vi "Create point.vi"(2 "Colour":T1={"Red"=1.0, "Green"=1.0, "Blue"=1.0, "Alpha"=1.0}, 3 "Point size":dbl=3.0, 4 "Point":sgl[](array[numeric])=[0.0, 0.0, 0.0]) -> (0 "Error out":errorcluster, 1 "Point out":refnum<vi>)   [LabVIEW 2017]
uses:
  <vilib>/Utility/miscctls.llb/LVRGBAColorTypeDef.ctl
  <vilib>/Utility/miscctls.llb/LV3DPointTypeDef.ctl
  <vilib>/picture/3D Picture Control/Object/Create Object (drawable).vi
  <vilib>/picture/3D Picture Control/NI_3D Picture Control.lvlib
panel:
  # "PN 23/10/17"
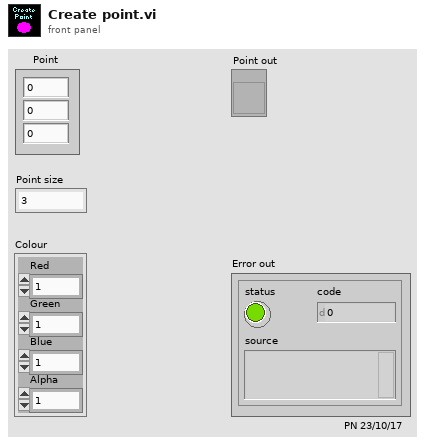
[diagram p1: front panel]
types:
  T1 = typedef "LVRGBAColorTypeDef.ctl" = cluster{"Red":sgl, "Green":sgl, "Blue":sgl, "Alpha":sgl}
  T2 = enum16{"Inherit Value", "Points", "Wireframe", "Polygons"}
  T3 = typedef "LV3DPointTypeDef.ctl" = cluster{"X":sgl, "Y":sgl, "Z":sgl}
  T4 = enum16{"Inherit Material", "Use entire Material", "Ignore Ambient", "Ignore Diffuse", "Ignore Specular", "Ignore Emission", "Ignore Ambient and Diffuse"}
  T5 = enum16{"Overall", "Per Primitive", "Per Vertex", "Binding Off"}
  T6 = enum16{"Points", "Lines", "Line Strip", "Line Loop", "Triangles", "Triangle Strip", "Triangle Fan", "Quads", "Quad Strip", "Polygon"}
  T7 = enum16{"Inherit Value", "No Culling", "Cull Back Face", "Cull Front Face", "Cull Both Faces"}
  T8 = enum16{"Inherit Value", "Counterclockwise", "Clockwise"}
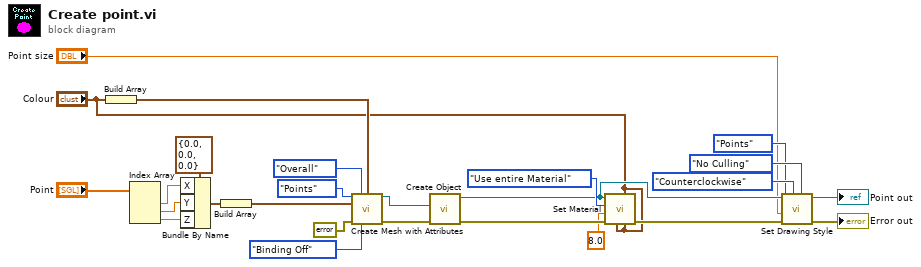
[diagram p0: block diagram]
diagram:
  n1 = Build Array("Colour") -> (w9:T1[])
  n2 = Index Array(array="Point") -> (element #1=w6:sgl, element #2=w5:sgl, element #3=w4:sgl)  [unwired: 3 in]
  n3 = Bundle By Name(cluster=T3 {"X"=0.0, "Y"=0.0, "Z"=0.0} ("3D Point"), "X"=w6, "Y"=w5, "Z"=w4) -> (w19:T3)
  n4 = Build Array(w19) -> (w2:T3[])
  n5 = call <vilib>:"Create Mesh with Attributes.vi"("Draw Mode"=T6."Points", "Color Binding Mode"=T5."Overall", "Color Array"=w9, "Vertex Array"=w2, "error in (no error)"=errorcluster {"status"=FALSE, "code"=0, "source"=""}, "Normal Binding Mode"=T5."Binding Off") -> ("New Mesh Refnum"=w21:refnum<vi>, "error out"=w22:errorcluster)  [unwired: 8 in]
  n6 = call-poly <vilib>:"Create Object.vi"("error in (no error)"=w22, "Geometry"=w21) -> ("error out"=w14:errorcluster, "Scene:New Object"=w10:refnum<vi>)  [unwired: 8 in]
  n7 = call <vilib>:"Set Material.vi"("Diffuse"="Colour", "Specular"="Colour", "Emission"="Colour", "error in (no error)"=w14, "Shininess"=sgl 8.0, "Color Mode"=T4."Use entire Material", "Scene Object In"=w10) -> ("error out"=w13:errorcluster)  [unwired: 3 in, 1 out]
  n8 = call <vilib>:"Set Drawing Style.vi"("Face Culling Mode"=T7."No Culling", "Frontface Mode"=T8."Counterclockwise", "error in (no error)"=w13, "Size"="Point size", "Mode"=T2."Points" ("Render mode"), "Scene Object In"=w10) -> ("error out"=→"Error out":errorcluster, "Scene Object Out"=→"Point out":refnum<vi>)  [unwired: 4 in]
